vi "DSC.Deregister.vi"(0 "HGF_DSCMonitor in":refnum<class "HGF_DSCMonitor.lvclass">, 1 "SV":refnum<k21>, 3 "HGF_NetworkVisitor":refnum<class "HGF_NetworkVisitor.lvclass">, 4 "Event Queue":refnum<queue>, 5 "error in (no error)":errorcluster, 9 "Switch":bool) -> (14 "HGF_DSCMonitor out":refnum<class "HGF_DSCMonitor.lvclass">, 19 "error out":errorcluster)   [LabVIEW 2009]
uses:
  HGF_DSCMonitor.lvclass
  HGF_BaseClasses/HGF_NetworkVisitor/HGF_NetworkVisitor.lvclass
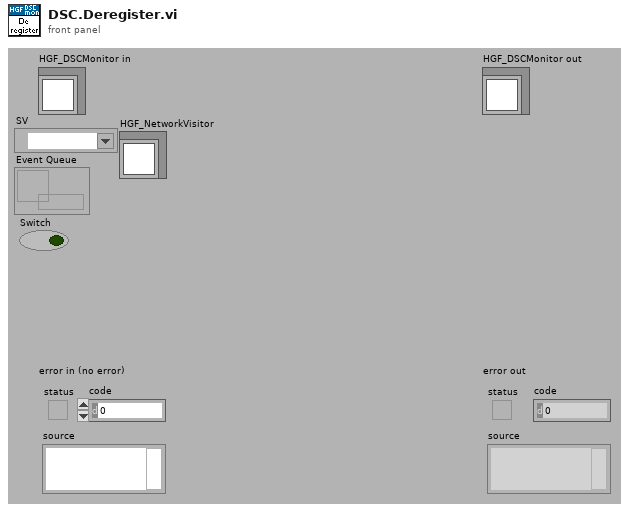
[diagram p1: front panel]
types:
  T1 = cluster{"Command":string, "SV":refnum<k21>, "HGF_NetworkVisitor":refnum<class "HGF_NetworkVisitor.lvclass">, "Event Queue":refnum<queue>, "request changes (all changes)":u16, "Switch":bool}
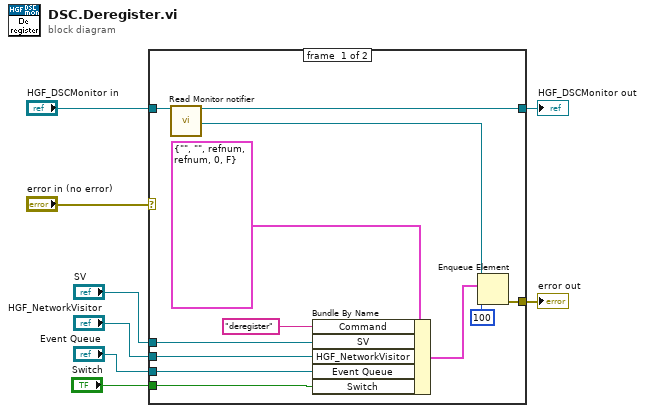
[diagram p0: block diagram]
diagram:
  n1 = case shown="No Error" "error in (no error)" {
    selector: "error in (no error)" -> [_ w22]
    tunnel: [w9 w22] -> w7
    tunnel: [w19 w21] -> w5
    tunnel: "HGF_DSCMonitor in" -> [w20 w21]
    tunnel: "SV" -> [w13 _]
    tunnel: "HGF_NetworkVisitor" -> [w12 _]
    tunnel: "Event Queue" -> [w11 _]
    tunnel: "Switch" -> [w10 _]
    frame #0 {
      n2 = call "Read Monitor notifier.vi"("HGF_DSCMonitor.lvclass in"=w20) -> ("HGF_DSCMonitor.lvclass out"=w19:refnum<class "HGF_DSCMonitor.lvclass">, "Monitor Queue"=w16:refnum<queue>)  [unwired: 2 in, 15 out]
      n3 = Bundle By Name(cluster=T1 {"Command"="", "SV"="", "HGF_NetworkVisitor"=refnum, "Event Queue"=refnum, "request changes (all changes)"=0, "Switch"=FALSE} ("element"), "Command"="deregister", "SV"=w13, "HGF_NetworkVisitor"=w12, "Event Queue"=w11, "Switch"=w10) -> (w17:T1)
      n4 = Enqueue Element(queue=w16, element=w17, timeout in ms (-1)=100) -> (error out=w9:errorcluster)  [unwired: 1 in, 2 out]
    }
    frame #1 {
    }
  }
  "error out" <- w7
  "HGF_DSCMonitor out" <- w5
